vi "Actor Core.vi"(8 "error in":errorcluster, 11 "Simulated User Console Actor in":refnum<class "Simulated Display Console Actor.lvclass">) -> (0 "error out":errorcluster, 3 "Actor out":refnum<class "Actor.lvclass">)   [LabVIEW 2019, in "Simulated Display Console Actor.lvlib" / "Simulated Display Console Actor.lvclass"]
doc: "(<B>Filename</B>: Actor Framework.lvlib:Actor.lvclass:Actor Core.vi)\n\nReceives messages to the actor, reacts to them, and initiates any error handling that may shut the actor down.\n\nDescendant classes may override this VI to append parallel tasks for the actor to complete while it handles messages. Overrides use the Call Parent Method node."
uses:
  Simulated Display Console Actor.lvclass
  C:/Program Files (x86)/National Instruments/LabVIEW 2019/vi.lib/ActorFramework/Actor/Actor.lvclass
  <vilib>/ActorFramework/Actor/Actor.lvclass
  <vilib>/ActorFramework/Actor/Actor.lvclass/Actor.ctl
  <vilib>/ActorFramework/Message Enqueuer/Message Enqueuer.lvclass/Message Enqueuer.ctl
  Simulated Display Console Actor.lvclass/Simulated Display Console Actor.ctl
  <vilib>/ActorFramework/Message Enqueuer/Init from Existing Queue.vi
  <vilib>/ActorFramework/Message Enqueuer/Enqueue.vi
  <vilib>/ActorFramework/Stop Msg/Stop Msg.lvclass
  C:/Program Files (x86)/National Instruments/LabVIEW 2019/vi.lib/ActorFramework/Message/Message.lvclass
  <vilib>/ActorFramework/Message Priority Queue/Priority Enqueue.vi
  Display Console/Display Console/Display Console Actor.lvclass
  <vilib>/ActorFramework/Message Enqueuer/Message Enqueuer.lvclass
panel:
  out "Card Read":bool
  out "Message Screen":string
  out "Current Transaction":string
  # "[Covers: UI3] \n[Covers: UI3A] \n[Covers: UI3B] \n[Covers: UI3C]"
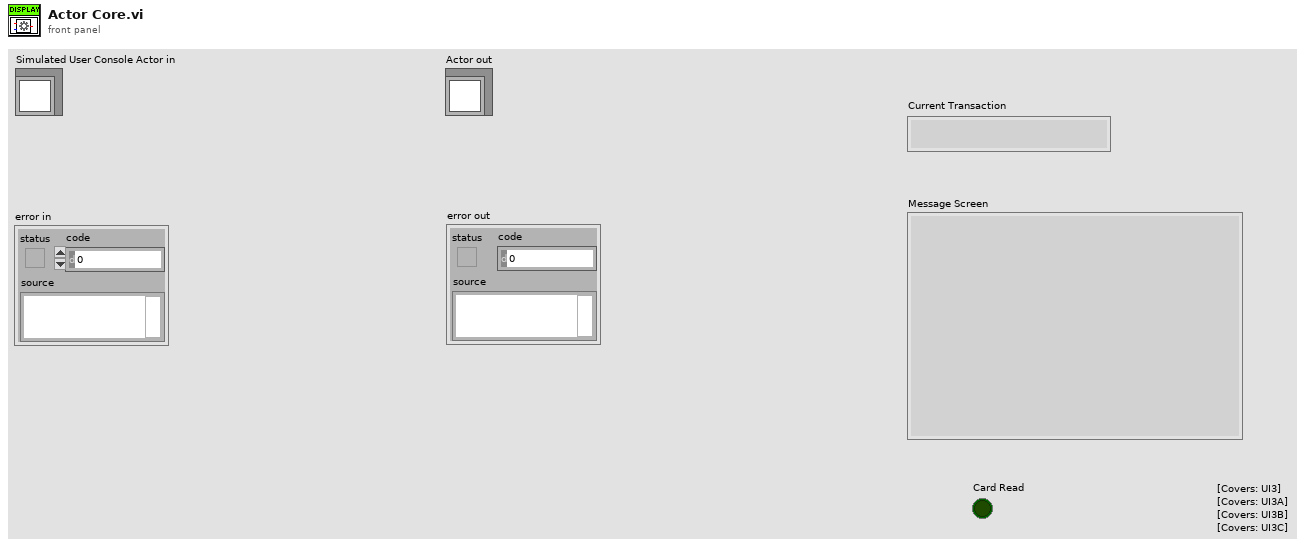
[diagram p1: front panel]
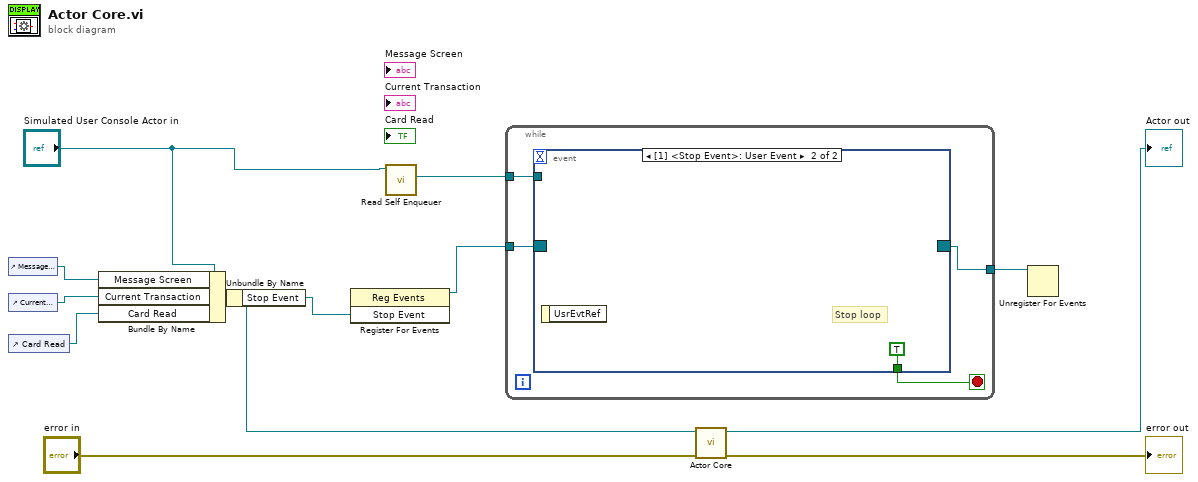
[diagram p0: block diagram]
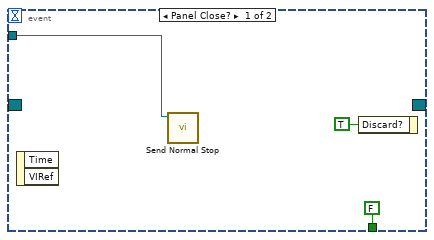
[diagram p2: hidden frame]
diagram:
  n1 = control-ref of="Message Screen"() -> (w3:refnum<vi>)
  n2 = control-ref of="Current Transaction"() -> (w2:refnum<vi>)
  n3 = control-ref of="Card Read"() -> (w1:refnum<vi>)
  n4 = Bundle By Name(cluster="Simulated User Console Actor in", "Message Screen"=w3, "Current Transaction"=w2, "Card Read"=w1) -> (w4:refnum<class "Simulated Display Console Actor.lvclass">)
  n5 = Unbundle By Name(w4) -> ("Stop Event"=w6:refnum<user-event>)
  n6 = register-events(w6) -> (reference out=w8:refnum<event-registration>)  [unwired: 2 in, 1 out]
  n7 = call <vilib>:"Read Self Enqueuer.vi"("Actor"="Simulated User Console Actor in") -> ("Self Enqueuer"=w9:refnum<class "Message Enqueuer.lvclass">)  [unwired: 10 in]
  n8 = while {
    tunnel: w9 -> [w15]
    tunnel: w8 -> [w14]
    tunnel: [w13] -> w7
    stop <- w16 stop-if-true
    n9 = event shown="[1] <Stop Event>: User Event" {
      selector: w14 -> [_ _]
      dyn-events: [_ _] -> w13
      timeout: _ -> [_ _]
      tunnel: [FALSE TRUE] -> w16
      tunnel: w15 -> [w18 _]
      event Panel Close? {
        n10 = event-data() -> ()  [unwired: 1 in, 2 out]
        n11 = call <vilib>:"Send Normal Stop.vi"("Message Enqueuer"=w18) -> ()  [unwired: 10 in, 1 out]
        n12 = event-data("Discard?"=TRUE) -> ()  [unwired: 1 in, 1 out]
      }
      event User Event {
        # "Stop loop"
        n13 = event-data() -> ()  [unwired: 1 in, 1 out]
      }
    }
  }
  n14 = call-parent "Actor Core.vi"("error in"="error in", "Actor in"=w4) -> ("error out"=→"error out":errorcluster, "Actor out"=→"Actor out":refnum<class "Actor.lvclass">)  [unwired: 8 in]
  n15 = Unregister For Events(event registration refnum=w7) -> ()  [unwired: 1 in, 1 out]
